vi "Create Event Log Title.vi"(8 "Event value":dbl, 9 "Actual value":dbl, 11 "Event name":T1) -> (1 "Threshold value":dbl, 3 "Log Title":string)   [LabVIEW 2024]
uses:
  Type Definitions/Threshold Events.ctl
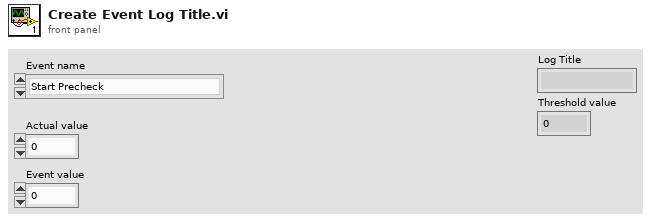
[diagram p1: front panel]
types:
  T1 = typedef "Threshold Events.ctl" = enum16{"Start Precheck", "Start Scenario", "Start Releasing", "Finish Releasing", "Clear Scenario", "Abort Scenario"}
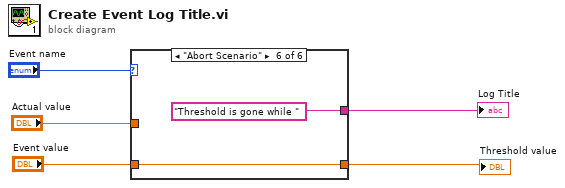
[diagram p0: block diagram]
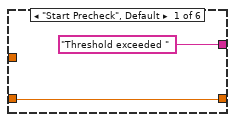
[diagram p2: hidden frame]
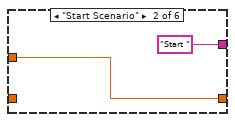
[diagram p3: hidden frame]
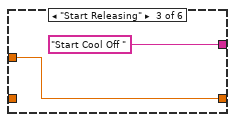
[diagram p4: hidden frame]
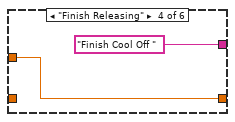
[diagram p5: hidden frame]
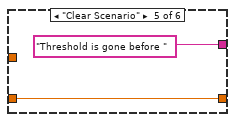
[diagram p6: hidden frame]
diagram:
  n1 = case shown="\"Abort Scenario\"" "Event name" {
    tunnel: ["Threshold exceeded " "Start " "Start Cool Off " "Finish Cool Off " "Threshold is gone before " "Threshold is gone while "] -> w4
    tunnel: "Event value" -> [w6 _ _ _ w14 w16]
    tunnel: [w6 w8 w10 w12 w14 w16] -> w3
    tunnel: "Actual value" -> [_ w8 w10 w12 _ _]
    frame "Start Precheck", Default {
    }
    frame "Start Scenario" {
    }
    frame "Start Releasing" {
    }
    frame "Finish Releasing" {
    }
    frame "Clear Scenario" {
    }
    frame "Abort Scenario" {
    }
  }
  "Log Title" <- w4
  "Threshold value" <- w3
